vi "Convert MultiSource Variant to Data [ColorFrame].vi"(8 "error in":errorcluster, 11 "MultiSource Variant":variant) -> (0 "error out":errorcluster, 3 "Byte Array":u8[](array[numeric]))   [LabVIEW 2014]
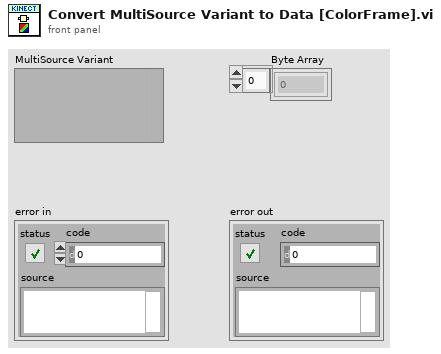
[diagram p1: front panel]
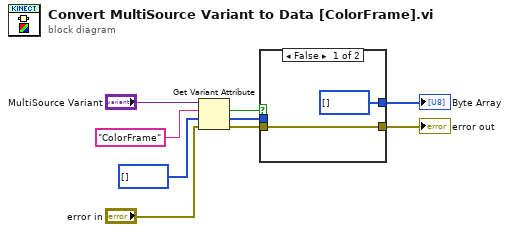
[diagram p0: block diagram]
diagram:
  n1 = Get Variant Attribute(Variant="MultiSource Variant", name="ColorFrame", default value (empty Variant)=u8[] [], error in="error in") -> (found=w2:bool, value=w5:u8[], error out=w6:errorcluster)  [unwired: 1 out]
  n2 = case shown="False" w2 {
    tunnel: w6 -> [w11 w13]
    tunnel: w5 -> [_ w12]
    tunnel: [w11 w13] -> w4
    tunnel: [u8[] [] w12] -> w3
    frame False {
    }
    frame True {
    }
  }
  "error out" <- w4
  "Byte Array" <- w3
